vi "Initialize.vi"(8 "error in (no error)":errorcluster, 10 "Path":path, 11 "Macro in":refnum<class "Macro.lvclass">) -> (0 "error out":errorcluster, 3 "Macro out":refnum<class "Macro.lvclass">)   [LabVIEW 2020, in "MacroAssert.lvlib" / "Macro.lvclass"]
uses:
  Macro.lvclass
  Macro.lvclass/Macro.ctl
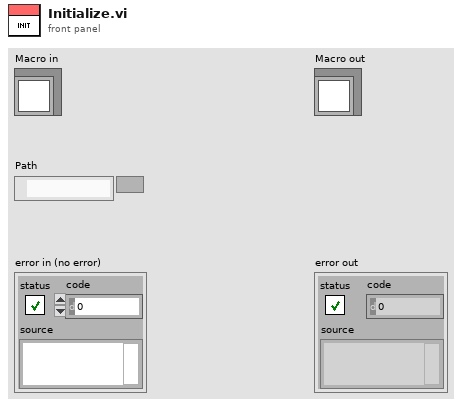
[diagram p1: front panel]
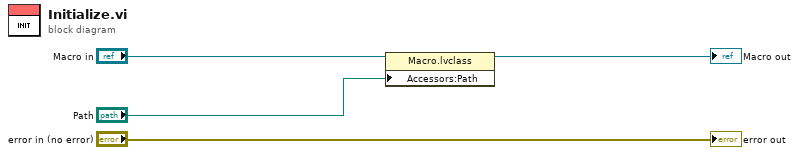
[diagram p0: block diagram]
diagram:
  n1 = property class="Macro.lvclass"(reference="Macro in", "Accessors:Path"="Path") -> (reference out=→"Macro out":refnum<class "Macro.lvclass">)  [unwired: 1 in, 1 out]
  "error out" <- "error in (no error)"
